vi "Write EndTime.vi"(8 "error in (no error)":errorcluster, 10 "EndTime":dbl, 11 "BaseWfrmPlugin in":refnum<class "BaseWfrmPlugin.lvclass">) -> (0 "error out":errorcluster, 3 "BaseWfrmPlugin out":refnum<class "BaseWfrmPlugin.lvclass">)   [LabVIEW 2014, in "WfrmPlugins.lvlib" / "BaseWfrmPlugin.lvclass"]
uses:
  BaseWfrmPlugin.lvclass
  BaseWfrmPlugin.lvclass/BaseWfrmPlugin.ctl
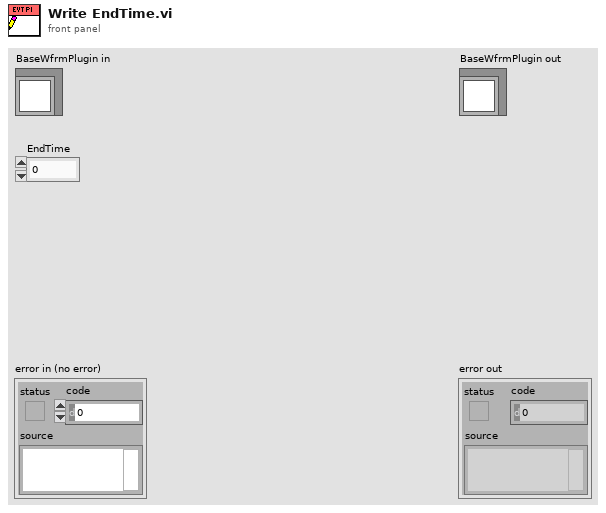
[diagram p1: front panel]
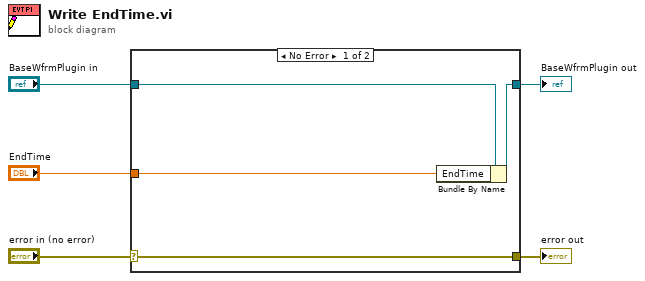
[diagram p0: block diagram]
diagram:
  n1 = case shown="No Error" "error in (no error)" {
    selector: "error in (no error)" -> [w9 w10]
    tunnel: [w9 w10] -> w4
    tunnel: [w7 w11] -> w2
    tunnel: "BaseWfrmPlugin in" -> [w8 w11]
    tunnel: "EndTime" -> [w6 _]
    frame No Error {
      n2 = Bundle By Name(cluster=w8, "EndTime"=w6) -> (w7:refnum<class "BaseWfrmPlugin.lvclass">)
    }
    frame Error {
    }
  }
  "error out" <- w4
  "BaseWfrmPlugin out" <- w2
